vi "Edgertronic-:get_storage_info copy.vi"(5 "Setup":T1={"URL"="130.64.16.195", "remote port"=80, "mode (standard)"=enum."Standard"}) -> (0 "error out":errorcluster, 1 "Storage Info:":T2={"Connection Information:"="", "Available Space"="20140911165611", "Mount Point"="20140911165611", "Storage Size"="20140911165611"}, 2 "data out":string="HTTP/1.0 200 OK\r\nContent-Type: text/html; charset=utf-8\r\nContent-Length: 313\r\nConnection: close\r\nDate: Tue, 16 Jun 2015 13:54:12 GMT\r\nServer: lighttpd/1.4.11 (edgertonic slow motion camera)\r\n\r\n{\"build_date\": \"20150112\", \"sw_build_date\": \"20140911165611\", \"fpga_initialized\": 1, \"hardware_revision\": 6, \"model_number\": 1, \"home_dir\": \"/home/root/ss-web\", \"ir_filter\": 1, \"mac_addr\": \"00:1B:C5:09:61:4D\", \"serial_console_enabled\": false, \"serial_number\": 333, \"fpga_version\": 70, \"hardware_configuration\": 1}")   [LabVIEW 2012]
doc: "This VI returns storage device information."
panel:
  in  "GET Cmd":string="/get_storage_info"
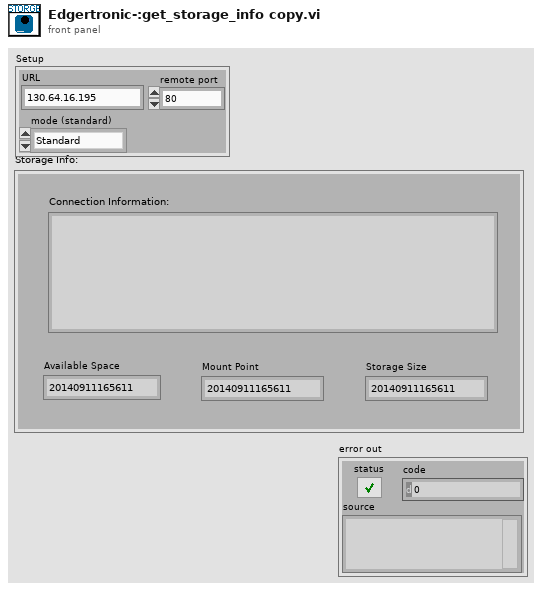
[diagram p1: front panel]
types:
  T1 = cluster{"URL":string, "remote port":u16, "mode (standard)":enum16{"Standard", "Buffered", "CRLF", "Immediate"}}
  T2 = cluster{"Connection Information:":string, "Available Space":string, "Mount Point":string, "Storage Size":string}
  T3 = cluster{"Parameter":string, "Parameter 2":string, "Parameter 3":string}
  T4 = cluster{"[0]":string, "[1]":string, "[2]":string, "[3]":string, "[4]":string, "[5]":string, "[6]":string, "[7]":string, "[8]":string}
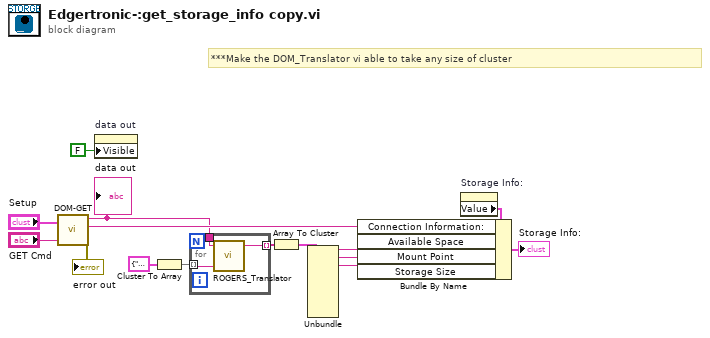
[diagram p0: block diagram]
diagram:
  # "***Make the DOM_Translator vi able to take any size of cluster"
  n1 = call <userlib>:"DOM-GET.vi"("Setup"="Setup", "GET Command"="GET Cmd") -> ("Data Out from Camera"=w7:string, "Connection Information"=w10:string, "error out"=→"error out":errorcluster)  [unwired: 1 out]
  "data out" <- w7
  n2 = property on="data out" class="Str"("Visible"=FALSE) -> ()  [unwired: 2 in, 2 out]
  n3 = Cluster To Array(cluster=T3 {"Parameter"="available_space", "Parameter 2"="mount_point", "Parameter 3"="storage_size"}) -> (array=w8:string[])
  n4 = for {
    tunnel: w8 -> [w16] mode=indexing
    tunnel: [w18] -> w1 mode=indexing
    tunnel: w7 -> [w17]
    n5 = call <userlib>:"ROGERS_Translator.vi"("Parameter"=w16, "data"=w17) -> ("String"=w18:string)  [unwired: 1 in, 2 out]
  }
  n6 = Array To Cluster(array=w1) -> (cluster=w6:T4)
  n7 = Unbundle(w6) -> ("[0]"=w5:string, "[1]"=w4:string, "[2]"=w3:string)  [unwired: 6 out]
  n8 = property on="Storage Info:" class="Clust (strict)"() -> ("Value"=w9:T2)  [unwired: 2 in, 2 out]
  n9 = Bundle By Name(cluster=w9, "Connection Information:"=w10, "Available Space"=w5, "Mount Point"=w4, "Storage Size"=w3) -> (→"Storage Info:":T2)
